vi "proc_format_error.vi"(0 "code in":i32) -> (1 "error":bool, 2 "code out":i32, 3 "error string":string)   [LabVIEW 2012]
doc: "Formats LV process error code into text."
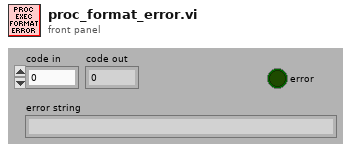
[diagram p1: front panel]
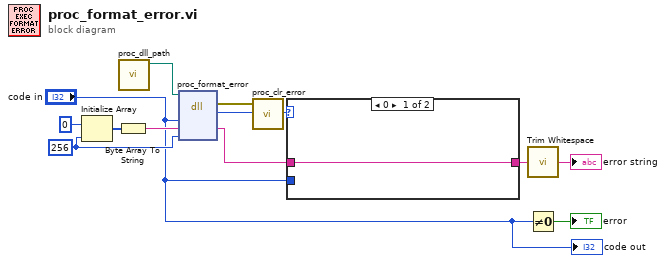
[diagram p0: block diagram]
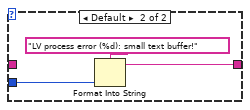
[diagram p2: hidden frame]
diagram:
  w7 = 256 ("dimension size")
  n1 = Initialize Array(u8 0 ("element"), w7) -> (w10:u8[])
  n2 = Byte Array To String(unsigned byte array=w10) -> (string=w9:string)
  n3 = call "proc_dll_path.vi"() -> ("path out"=w12:path)  [unwired: 10 in, 1 out]
  n4 = dll-call lib="lv_proc.dll" fn="proc_format_error"(path in=w12, "code"="code in", "buffer"=w9, "len"=w7) -> (error out=w11:errorcluster, "error"=w6:i32, "buffer"=w5:string)  [unwired: 4 in, 1 out]
  n5 = call "proc_clr_error.vi"("error in (no error)"=w11) -> ()  [unwired: 4 in, 1 out]
  n6 = case shown="0" w6 {
    tunnel: w5 -> [w13 _]
    tunnel: "code in" -> [_ w16]
    tunnel: [w13 w14] -> w4
    frame 0 {
    }
    frame Default {
      n7 = Format Into String(format string="LV process error (%d): small text buffer!", w16) -> (resulting string=w14:string)  [unwired: 2 in, 1 out]
    }
  }
  n8 = call <vilib>:"Trim Whitespace.vi"("string"=w4) -> ("trimmed string"=→"error string":string)  [unwired: 1 in]
  n9 = Not Equal To 0?(x="code in") -> (x != 0?=→"error":bool)
  "code out" <- "code in"
